vi "orderAnalysis.vi"(8 "ErrorIn":errorcluster, 10 "Tacho signal In":waveform(dbl), 11 "AccelerationDataIn":waveform(dbl)[](array[waveform])) -> (0 "ErrorOut":errorcluster, 1 "Orders and indicators":T1[](array[typedef]), 2 "Rotational speed [RPM]":dbl format="%0.2f", 3 "order power spectra":T2(array[cluster]) {"order 0" format="%.2p"; "delta order" format="%.2p"; "magnitude" format="%.2f"})   [LabVIEW 2019]
uses:
  OrderAndIndicators.ctl
  <vilib>/addons/Sound and Vibration/svt_Calibration/SVL Scale Voltage to EU (1 Ch).vi
  <vilib>/addons/Sound and Vibration/svt_Calibration/SVL Scale Voltage to EU (N Ch - 1 Info).vi
  <vilib>/Analysis/baseanly.llb/Mean (DBL).vi
  <vilib>/addons/_NISVFA/_Spectrum Processing/SVFA Power in Band (N Ch).vi
  <vilib>/addons/_NISVFA/_Shared subVIs/Common/svc_Set SV Channel Info.vi
  <vilib>/addons/_NISVFA/_Spectrum Processing/SVFA Power in Band (1 Ch).vi
  <vilib>/addons/_NISVFA/_Shared subVIs/Common/svc_Set SV Channel Info (variant).vi
  <vilib>/addons/_NISVFA/_Spectrum Processing/SVFA Get Spectrum Subset.vi
  <vilib>/addons/_NISVFA/_Spectrum Processing/SVFA Get Spectrum Subset (1 Ch).vi
  <vilib>/addons/_NISVFA/_Shared subVIs/Common/svc_Spectrum Units.vi
  <vilib>/addons/_NISVFA/_Spectrum Processing/SVFA Unit Conversion.vi
  <vilib>/addons/_NISVFA/_Spectrum Processing/SVFA Unit Conversion (1 Ch).vi
  <vilib>/addons/_NISVFA/_Shared subVIs/Common/SVL Set dB Reference (variant).vi
  <vilib>/dlg_ctls.llb/Space Constant.vi
  <vilib>/addons/_NISVFA/_Spectrum Processing/subVIs/svfa_Conversion Utility (spectrum info).vi
  <vilib>/addons/_NISVFA/_Spectrum Processing/subVIs/svfa_Peak to RMS to Peak2Peak.vi
  <vilib>/addons/_NISVFA/_Spectrum Processing/subVIs/svfa_Mag to Mag2.vi
  <vilib>/addons/_NISVFA/_Spectrum Processing/subVIs/svfa_Linear to dB.vi
  <vilib>/addons/_NISVFA/_Spectrum Processing/subVIs/svfa_dBrefA to dBrefB.vi
  <vilib>/addons/_NISVFA/_Spectrum Processing/subVIs/svfa_Spectrum to Spectral Density.vi
  <vilib>/Waveform/WDTOps.llb/WDT Waveform Duration DBL.vi
  <vilib>/Waveform/WDTOps.llb/WDT Get Waveform Subset DBL.vi
  <vilib>/addons/_NISVFA/_Shared subVIs/Common/svc_Engineering Units to Unit Label.vi
  <vilib>/addons/_NISVFA/_Shared subVIs/Common/svc_Compute Scale Factor to Convert V to EU.vi
  <vilib>/addons/_NISVFA/_Shared subVIs/Common/svc_Compute Scale Factor to Convert C to EU.vi
  <vilib>/addons/_NISVFA/_Shared subVIs/Common/svc_Set dB ref if Pascal.vi
  <vilib>/addons/_NISVFA/_Shared subVIs/Common/svc_Caller VI Returned in Error Source.vi
  <vilib>/addons/Sound and Vibration/Order Analysis/Tach Process/OAT Analog Tacho Process (1 Tacho).vi
  <vilib>/addons/Sound and Vibration/Order Analysis/Resample Order Tracking/OAT Convert to Even Angle Signal (N Channels).vi
  <vilib>/addons/Sound and Vibration/Order Analysis/Resample Order Tracking/OAT Order Power Spectrum (N Channels).vi
  <vilib>/addons/_NISVFA/_Shared subVIs/Common/svc_Format Value (DBL).vi
  <vilib>/addons/_NISVFA/_Shared subVIs/Common/svc_Surround NonAlpha String with Parentheses.vi
  <vilib>/addons/_NISVFA/_Shared subVIs/Common/svc_Get Weighting Enum and Labels.vi
  <vilib>/addons/_NISVFA/_Shared subVIs/Common/svc_Check Frequency Range in Spectrum.vi
  <vilib>/addons/_NISVFA/_Shared subVIs/Common/svc_Convert Frequency to Frequency String.vi
  <vilib>/addons/_NISVFA/_Shared subVIs/Common/svc_Build Unit Label for Frequency Range.vi
  <vilib>/addons/_NISVFA/_Shared subVIs/Common/svc_Window Parameters.vi
  <vilib>/addons/_NISVFA/_Spectrum Processing/subVIs/svfa_Spectrum Info Window to windowTd Type Def.vi
  <vilib>/addons/Sound and Vibration/Order Analysis/Tach Process/SoundVib_TachProcess.lvlib
  <vilib>/addons/Sound and Vibration/Order Analysis/Resample Order Tracking/SoundVib_OrderTracking.lvlib
  <vilib>/addons/Sound and Vibration/svt_Calibration/SoundVib_Calibration.lvlib
  <vilib>/Analysis/NI_AALBase.lvlib
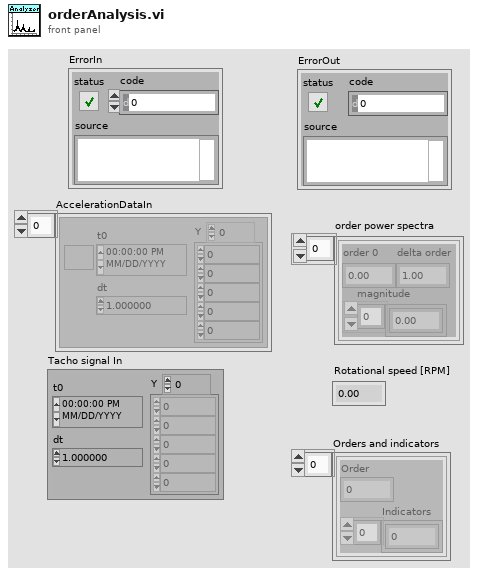
[diagram p1: front panel]
types:
  T1 = typedef "OrderAndIndicators.ctl" = cluster{"Order":dbl, "Indicators":dbl[]}
  T2 = cluster{"order 0":dbl, "delta order":dbl, "magnitude":dbl[]}[]
  T3 = typedef "AnalyzerSettings.ctl" = cluster{"Create NS Timeout Code":i32, "Destroy NS Timeout Code":i32, "All threads":T4[], "Connected to app?":bool, "AnalysisSettings":T5}
  T4 = typedef "AThreads.ctl" = enum16{"UI", "analyzeAccelerationData", "aquireAccelerationData", "communicateWebServices", "TDMSmanager", "aquireTachoSignal"}
  T5 = typedef "AnalysisSettings.ctl" = cluster{"Fault Thresholds":T6, "Analysis series name":string, "Save data analysis?":bool, "Band size":i32, "OrderAnalysis?":bool, "Accelerometer":T8, "fs [Hz]":dbl, "Pulse per revolution":u16}
  T6 = typedef "Thresholds.ctl" = cluster{"Parameters labels":T7[], "Parameters thresholds":dbl[], "Freqs and thresholds":dbl[][], "Orders and thresholds":dbl[][]}
  T7 = typedef "FaultParameter.ctl" = enum16{"Kurtosis", "RMS", "Crest factor"}
  T8 = typedef "Accelerometer.ctl" = enum16{"None", "MPU6050", "MMA7351"}
  T9 = typedef "SoundVib_TachProcess.lvlib/speed profile.ctl" = cluster{"time [s]":dbl[], "speed [RPM]":dbl[]}
  T10 = typedef "svc_Resampled Channel Info.ctl" = cluster{"channel name":string, "description":string, " channel info":T11}
  T11 = typedef "svc_Channel Info.ctl" = cluster{"sensor sensitivity":dbl, "engineering units":T12, "dB reference":dbl, "custom label":string, "weighting filter":T13, "pregain":dbl}
  T12 = typedef "svc_Engineering Units Text Ring.ctl" = u16
  T13 = typedef "svc_Weighting Filter Text Ring.ctl" = u16
  T14 = typedef "svc_Spectrum Info.ctl" = cluster{"channel name":string, "description":string, "x-axis units":T15, "spectral info":cluster{"spectrum type":T16, "linear/dB":enum16{"linear", "dB"}, "window":u16, "window size":i32, "FFT size":i32}, "engineering units":T12, "custom label":string, "dB reference [EU]":dbl, "peak units":enum16{"rms", "peak", "peak-peak"}, "weighting filter":T13, "spectral density?":bool, "unit label":string, "spectrum skewed?":bool, "complimentary spectrum units":T17}
  T15 = typedef "svc_X-Axis Units.ctl" = u16
  T16 = typedef "svc_Spectrum Type.ctl" = enum16{"FFT Spectrum [complex]", "Amplitude [Magnitude]", "Power [Magnitude^2]", "Cross Spectrum [complex]", "Frequency Response [Complex]"}
  T17 = typedef "svc_Complimentary Spectrum Units.ctl" = enum16{"none", "radians", "degrees", "cycles", "imaginary"}
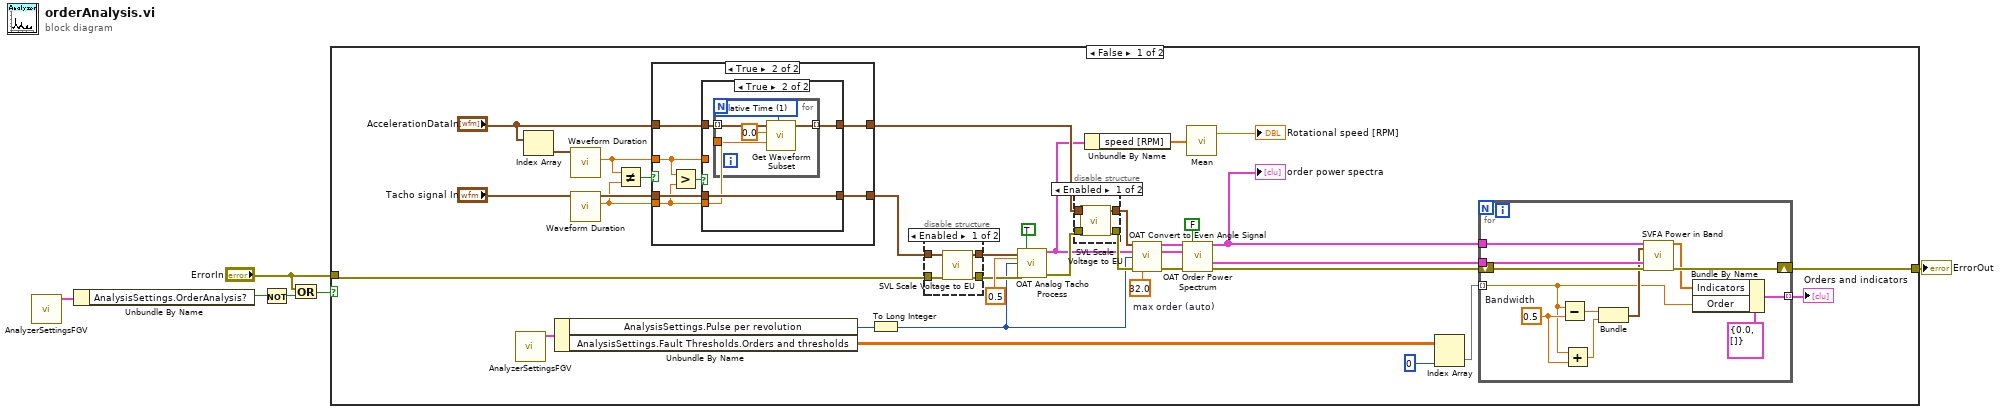
[diagram p0: block diagram]
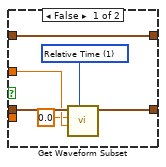
[diagram p5: hidden frame]
diagram:
  n1 = call "AnalyzerSettingsFGV.vi"() -> ("AnalyzerSettingsOut"=w5:T3)  [unwired: 11 in]
  n2 = Unbundle By Name(w5) -> ("AnalysisSettings.OrderAnalysis?"=w4:bool)
  n3 = Not(x=w4) -> (.not. x?=w3:bool)
  n4 = Or(x="ErrorIn", y=w3) -> (x .or. y?=w2:bool)
  n5 = case shown="False" w2 {
    tunnel: [w18 w91] -> w6
    tunnel: "ErrorIn" -> [w27 w91]
    frame False {
      w22 = 32.0  # max order (auto)
      n6 = call "AnalyzerSettingsFGV.vi"() -> ("AnalyzerSettingsOut"=w26:T3)  [unwired: 11 in]
      n7 = Index Array(array="AccelerationDataIn") -> (element=w39:waveform(dbl))  [unwired: 1 in]
      n8 = Unbundle By Name(w26) -> ("AnalysisSettings.Pulse per revolution"=w8:u16, "AnalysisSettings.Fault Thresholds.Orders and thresholds"=w25:dbl[][])
      n9 = call-poly <vilib>:"Waveform Duration.vi"("waveform in"=w39) -> ("duration"=w34:dbl)  [unwired: 8 in, 2 out]
      n10 = call-poly <vilib>:"Waveform Duration.vi"("waveform in"="Tacho signal In") -> ("duration"=w33:dbl, "waveform out"=w35:waveform(dbl))  [unwired: 8 in, 1 out]
      n11 = Not Equal?(x=w34, y=w33) -> (x != y?=w37:bool)
      n12 = case shown="True" w37 {
        tunnel: "AccelerationDataIn" -> [w68 w73]
        tunnel: w35 -> [w67 w74]
        tunnel: [w68 w69] -> w14
        tunnel: [w67 w70] -> w28
        tunnel: w34 -> [_ w72]
        tunnel: w33 -> [_ w71]
        frame False {
        }
        frame True {
          n13 = Greater?(x=w72, y=w71) -> (0:w75:bool)
          n14 = case shown="True" w75 {
            tunnel: w74 -> [w81 w85]
            tunnel: w73 -> [w78 w84]
            tunnel: w72 -> [w80 _]
            tunnel: w71 -> [_ w83]
            tunnel: [w79 w85] -> w70
            tunnel: [w78 w82] -> w69
            frame False {
              w76 = u16 1 items=["Samples", "Relative Time"] ("start/duration format")
              n15 = call-poly <vilib>:"Get Waveform Subset.vi"("start/duration format"=w76, "duration"=w80, "start samples/time"=0.0, "waveform in"=w81) -> ("waveform out"=w79:waveform(dbl))  [unwired: 2 in, 3 out]
            }
            frame True {
              n16 = for {
                tunnel: w84 -> [w90] mode=indexing
                tunnel: w83 -> [w89]
                tunnel: [w88] -> w82 mode=indexing
                w86 = u16 1 items=["Samples", "Relative Time"] ("start/duration format")
                n17 = call-poly <vilib>:"Get Waveform Subset.vi"("start/duration format"=w86, "duration"=w89, "start samples/time"=0.0, "waveform in"=w90) -> ("waveform out"=w88:waveform(dbl))  [unwired: 2 in, 3 out]
              }
            }
          }
        }
      }
      n18 = To Long Integer(number=w8) -> (32bit integer=w7:i32)
      n19 = disable-structure shown="Enabled" {
        disable-tunnel: [w52 w54] -> w30
        disable-tunnel: [w51 w53] -> w29
        disable-tunnel: w28 -> [w50 w54]
        disable-tunnel: w27 -> [w49 w53]
        frame Enabled {
          n20 = call-poly <vilib>:"SVL Scale Voltage to EU.vi"("error in (no error)"=w49, "signal [V]"=w50) -> ("error out"=w51:errorcluster, "scaled signal [EU]"=w52:waveform(dbl))  [unwired: 7 in, 1 out]
        }
        frame Disabled {
        }
      }
      n21 = call-poly <vilib>:"OAT Analog Tacho Process.vi"("analog tacho signal"=w30, "missing pulses? (no:F)"=TRUE, "threshold (auto)"=0.5, "pulse/revolution (1)"=w7, "error in (no error)"=w29) -> ("speed profile"=w11:T9, "error out"=w13:errorcluster)  [unwired: 6 in, 3 out]
      n22 = disable-structure shown="Enabled" {
        disable-tunnel: [w46 w48] -> w15
        disable-tunnel: w14 -> [w45 w48]
        disable-tunnel: w13 -> [w44 w47]
        disable-tunnel: [w43 w47] -> w12
        frame Enabled {
          n23 = call-poly <vilib>:"SVL Scale Voltage to EU.vi"("error in (no error)"=w44, "signals [V]"=w45) -> ("error out"=w43:errorcluster, "scaled signals [EU]"=w46:waveform(dbl)[])  [unwired: 7 in, 1 out]
        }
        frame Disabled {
        }
      }
      n24 = Unbundle By Name(w11) -> ("speed [RPM]"=w10:dbl[])
      n25 = call-poly <vilib>:"OAT Convert to Even Angle Signal.vi"("scaled signals [EU]"=w15, "speed profile"=w11, "pulse/revolution (1)"=w7, "error in (no error)"=w12, "max order (auto)"=w22) -> ("even-angle signals"=w23:cluster{"r0":dbl, "dr":dbl, "Y":dbl[]}[], "even-angle channel info"=w41:T10[], "error out"=w42:errorcluster)  [unwired: 6 in, 2 out]
      n26 = call-poly <vilib>:"OAT Order Power Spectrum.vi"("even-angle signals"=w23, "dB on? (T)"=FALSE, "even-angle channel info"=w41, "error in (no error)"=w42) -> ("order power spectra"=w20:T2, "spectrum info"=w19:T14[], "error out"=w21:errorcluster)  [unwired: 5 in, 4 out]
      "order power spectra" <- w20
      n27 = call-poly <vilib>:"Mean.vi"("X"=w10) -> ("mean"=→"Rotational speed [RPM]":dbl)  [unwired: 1 out]
      n28 = Index Array(array=w25, index (col)=0 ("disabled index (col)")) -> (element=w17:dbl[])  [unwired: 1 in]
      n29 = for {
        tunnel: w20 -> [w63]
        tunnel: w19 -> [w65]
        shift-right: [w64] -> w18
        shift-left: w21 -> [w66]
        tunnel: w17 -> [w56] mode=indexing
        tunnel: [w55] -> w16 mode=indexing
        w62 = 0.5  # Bandwidth
        n30 = Subtract(x=w56, y=w62) -> (x-y=w61:dbl)
        n31 = Add(x=w56, y=w62) -> (x+y=w60:dbl)
        n32 = Bundle(w61, w60) -> (w59:cluster{dbl, dbl})  [unwired: 1 in]
        n33 = call-poly <vilib>:"SVFA Power in Band.vi"("spectra"=w63, "range"=w59, "spectrum info"=w65, "error in (no error)"=w66) -> ("powers in band"=w57:dbl[], "error out"=w64:errorcluster)  [unwired: 13 in, 1 out]
        n34 = Bundle By Name(cluster=T1 {"Order"=0.0, "Indicators"=[]} ("Order and indicators"), "Indicators"=w57, "Order"=w56) -> (w55:T1)
      }
      "Orders and indicators" <- w16
    }
    frame True {
    }
  }
  "ErrorOut" <- w6
